vi "random_number_generator.vi"() -> ()   [LabVIEW 2014]
uses:
  <vilib>/imath/engines/lvmath2/RunTimeEngine/Managers/WorkSpace/UID Generator.vi
  <vilib>/imath/engines/lvmath2/RunTimeEngine/BuiltInFunctions/randint/NIMS_randint(1,1,RV).vi
  <vilib>/imath/engines/lvmath2/RunTimeEngine/RunTimeType/NIMS_RunTimeType_From StrictType (excl LVString).vi
  <instcachedir>/0/NIMS_RunTimeType_From StrictType (excl LVString)_15A5391EEA9C4AACB9955AC755B83D29.lvgen/NIMS_RunTimeType_From StrictType (excl LVString)_15A5391EEA9C4AACB9955AC755B83D29_000.vi
  <vilib>/imath/engines/lvmath2/RunTimeEngine/RunTimeType/NIMS_RunTimeType_Set Source Original Bool.vi
  <vilib>/imath/engines/lvmath2/RunTimeEngine/ErrorHandling/NIMS_Create Error From Enums.vi
  <vilib>/imath/engines/lvmath2/RunTimeEngine/LocalVariableDefStatement/MC_LocalVariableDefStatement_Display.vi
  <vilib>/imath/engines/lvmath2/RunTimeEngine/BuiltInFunctions/rand/NIMS_rand().vi
  <vilib>/imath/engines/lvmath2/RunTimeEngine/ErrorHandling/NIMS_Error From Error Code.vi
  <vilib>/imath/engines/lvmath2/RunTimeEngine/Managers/SymbolTable/Clear UID.vi
  <vilib>/imath/engines/lvmath2/RunTimeEngine/NodeEndStatement/NIMS_NodeEndStatement_Output.vi
  <instcachedir>/0/NIMS_NodeEndStatement_Output_53EC0D466D134D7ABD903AC30B43404B.lvgen/NIMS_NodeEndStatement_Output_53EC0D466D134D7ABD903AC30B43404B_001.vi
  <instcachedir>/0/NIMS_NodeEndStatement_Output_53EC0D466D134D7ABD903AC30B43404B.lvgen/NIMS_NodeEndStatement_Output_53EC0D466D134D7ABD903AC30B43404B_015.vi
  <vilib>/imath/engines/lvmath2/RunTimeEngine/ErrorHandling/NIMS_Finalize Error.vi
  <vilib>/imath/engines/lvmath2/RunTimeEngine/Managers/SymbolTable/NIMS_WorkSpace.lvlib
panel:
  out "Array 3":dbl[][](array[numeric])
  out "Array 2":dbl[][](array[numeric])
  out "Array":bool[][](array[boolean])
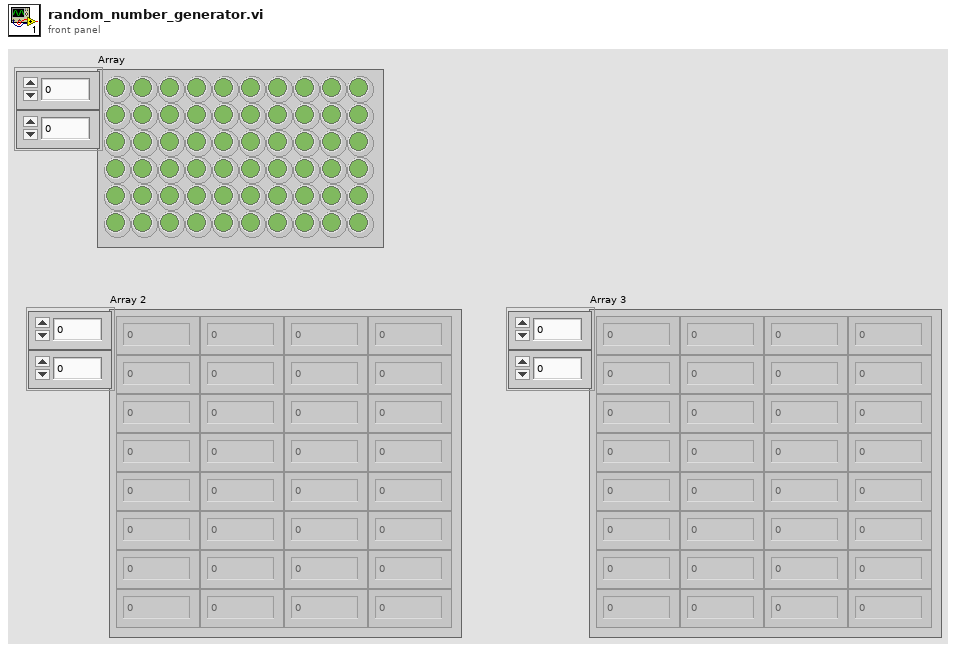
[diagram p1: front panel]
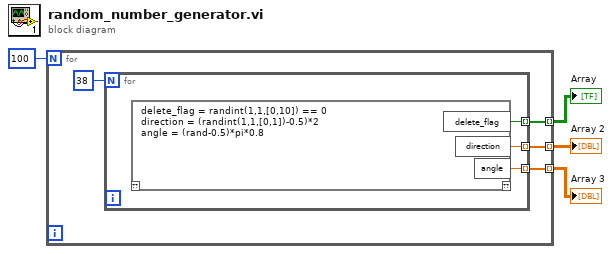
[diagram p0: block diagram]
diagram:
  n1 = for {
    N: 100 -> [_]
    tunnel: [w7] -> w3 mode=indexing
    tunnel: [w6] -> w2 mode=indexing
    tunnel: [w5] -> w1 mode=indexing
    n2 = for {
      N: 38 -> [_]
      tunnel: [w11] -> w7 mode=indexing
      tunnel: [w10] -> w6 mode=indexing
      tunnel: [w9] -> w5 mode=indexing
      n3 = mathscript code="delete_flag = randint(1,1,[0,10]) == 0\ndirection = (randint(1,1,[0,1])-0.5)*2\nangle = (rand-0.5)*pi*0.8"() -> ("delete_flag"=w11:bool, "direction"=w10:dbl, "angle"=w9:dbl)  [unwired: 1 in, 1 out]
    }
  }
  "Array" <- w3
  "Array 2" <- w2
  "Array 3" <- w1
